vi "ConfirmApprovedList.vi"(8 "error in (no error)":errorcluster, 11 "ApprovedDeps":T2[](array[typedef])) -> (0 "error out":errorcluster, 2 "Update?":bool, 3 "Confirmed Deps List":T1[](array[typedef]))   [LabVIEW 2019, in "Hawkeye.lvlib"]
uses:
  Hawkeye.lvlib
  Typedefs/ApprovedDeps.ctl
  Typedefs/ConfirmDeps.ctl
panel:
  out "No of .Hawkeyes to update":i32
  out "No change":enum8{"False", "True", "Mixed"}(c332)
  out "Remove from .Hawkeye":enum8{"False", "True", "Mixed"}(c332)=enum."Mixed"
  out "Add to .Hawkeye":enum8{"False", "True", "Mixed"}(c332)=enum."True"
  in  "Cancel?":bool
  in  "Ok?":bool
  # ".Hawkeye Update Status"
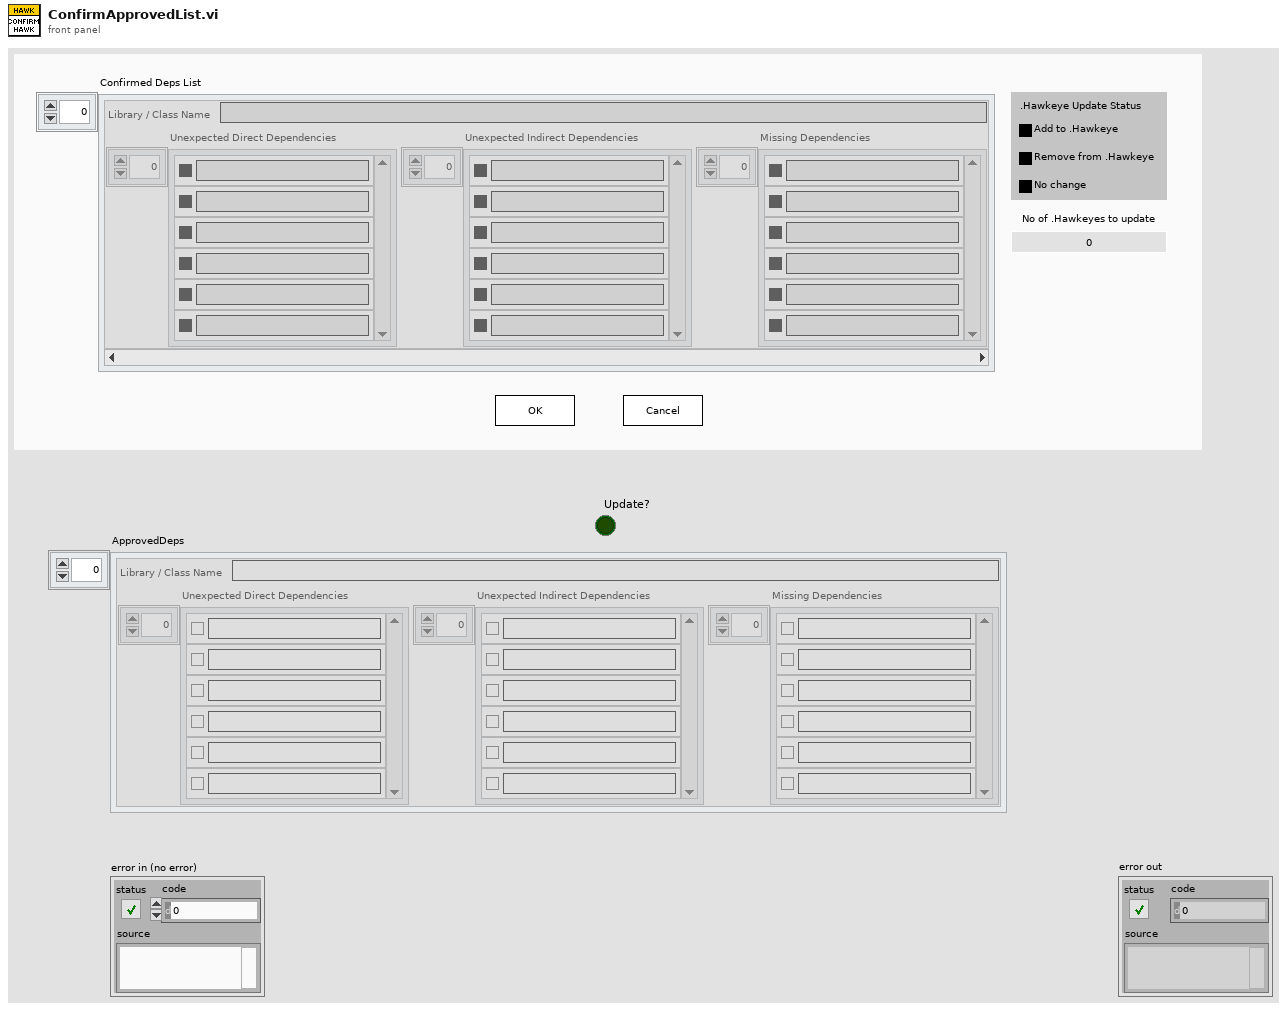
[diagram p1: front panel]
types:
  T1 = typedef "Hawkeye.lvlib/ConfirmDeps.ctl" = cluster{"Library / Class Name":string, "Unexpected Direct Dependencies":cluster{"Confirm Status":enum8{"False", "True", "Mixed"}, "Library / Class Name":string}[], "Unexpected Indirect Dependencies":cluster{"Confirm Status":enum8{"False", "True", "Mixed"}, "Library / Class Name":string}[], "Missing Dependencies":cluster{"Confirm Status":enum8{"False", "True", "Mixed"}, "Library / Class Name":string}[]}
  T2 = typedef "Hawkeye.lvlib/ApprovedDeps.ctl" = cluster{"Library / Class Name":string, "Unexpected Direct Dependencies":cluster{"Approved":bool, "Library / Class Name":string}[], "Unexpected Indirect Dependencies":cluster{"Approved":bool, "Library / Class Name":string}[], "Missing Dependencies":cluster{"Approved":bool, "Library / Class Name":string}[]}
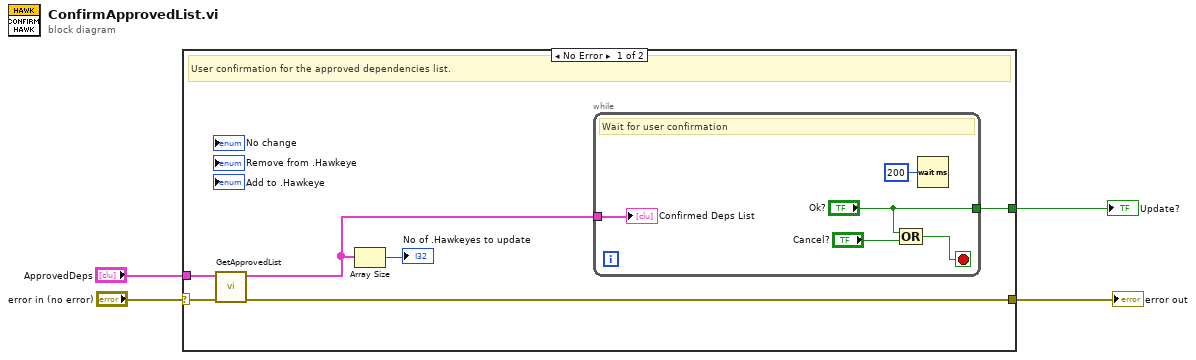
[diagram p0: block diagram]
diagram:
  n1 = case shown="No Error" "error in (no error)" {
    selector: "error in (no error)" -> [w8 w16]
    tunnel: [w7 w16] -> w3
    tunnel: "ApprovedDeps" -> [w9 _]
    tunnel: [w10 _] -> w1
    frame No Error {
      # "User confirmation for the approved dependencies list."
      n2 = call "GetApprovedList.vi"("error in (no error)"=w8, "ApprovedDeps"=w9) -> ("error out"=w7:errorcluster, "Confirmed Deps List"=w6:T1[])  [unwired: 8 in]
      n3 = Array Size(array=w6) -> (size(s)=→"No of .Hawkeyes to update":i32)
      n4 = while {
        tunnel: ["Ok?"] -> w10
        tunnel: w6 -> [w11]
        stop <- w13 stop-if-true
        # "Wait for user confirmation"
        n5 = Compound Arithmetic op=OR("Ok?", "Cancel?") -> (w13:bool)
        n6 = Wait (ms)(milliseconds to wait=u32 200) -> ()  [unwired: 1 out]
        "Confirmed Deps List" <- w11
      }
    }
    frame Error {
    }
  }
  "error out" <- w3
  "Update?" <- w1
